vi "GFGmultipleSet.vi"(8 "error in (no error)":errorcluster, 9 "Source VI":string, 11 "Array of Clusters of Variables":T2(array[cluster])) -> (0 "error out":errorcluster)   [LabVIEW 2012, in "GFG library.lvlib"]
doc: "SciScan 1.2 160622"
uses:
  GFG library.lvlib
  <vilib>/Utility/VariantDataType/Type.ctl
  <vilib>/Utility/VariantDataType/VariantType.lvlib
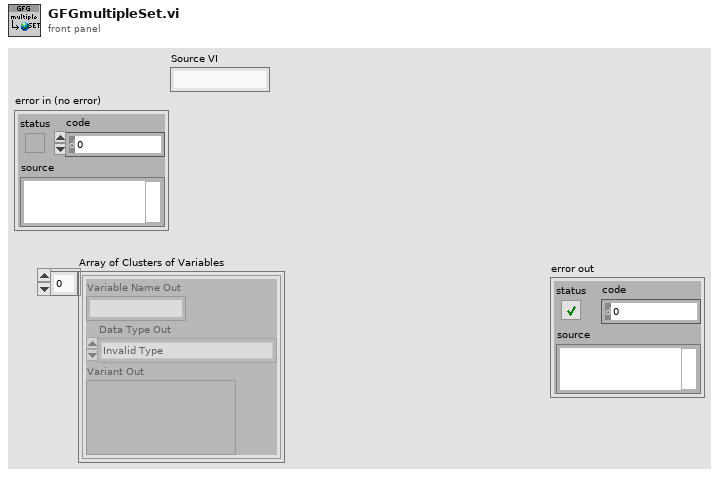
[diagram p1: front panel]
types:
  T1 = typedef "VariantType.lvlib/Type.ctl" = enum8{"Invalid Type", "Void", "I8", "I16", "I32", "I64", "U8", "U16", "U32", "U64", "Single Float", "Double Float", "Extended Float", "Single Complex", "Double Complex", "Extended Complex", "Enum U8", "Enum U16", "Enum U32", "Enum U64", "Single Float With Unit", "Double Float With Unit", "Extended Float With Unit", "Single Complex with Unit", "Double Complex with Unit", "Extended Complex with Unit", "Boolean", "String", "Path", "Picture", "Tag", "Array", "Cluster", "Variant", "LV Variant", "Waveform", "Timestamp", "Digital Waveform", "Digital Data", "ExpressData", "Refnum", "External Data", "VI", "Poly VI", "LabVIEW Class Instance", "Fixed Point"}
  T2 = cluster{"Variable Name Out":string, "Data Type Out":T1, "Variant Out":variant}[]
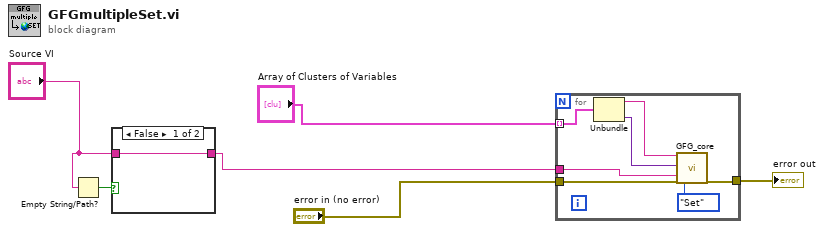
[diagram p0: block diagram]
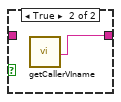
[diagram p2: hidden frame]
diagram:
  n1 = Empty String/Path?(string/path="Source VI") -> (empty?=w3:bool)
  n2 = case shown="False" w3 {
    tunnel: [w7 w8] -> w1
    tunnel: "Source VI" -> [w7 _]
    frame False {
    }
    frame True {
      n3 = call "getCallerVIname.vi"() -> ("VI name"=w8:string)  [unwired: 19 in]
    }
  }
  n4 = for {
    tunnel: [w14] -> w4
    tunnel: "Array of Clusters of Variables" -> [w13] mode=indexing
    tunnel: w1 -> [w10]
    tunnel: "error in (no error)" -> [w9]
    n5 = Unbundle(w13) -> ("Variable Name Out"=w12:string, "Variant Out"=w11:variant)  [unwired: 1 out]
    n6 = call "GFG_core.vi"("Variable Name in"=w12, "Variant in"=w11, "Source VI"=w10, "error in (no error)"=w9, "Action"=enum16{"Init", "Set", "Get"}."Set") -> ("error out"=w14:errorcluster)  [unwired: 8 in, 6 out]
  }
  "error out" <- w4
